vi "ReadHighTemp.vi"(8 "error in (no error)":errorcluster) -> (0 "error out":errorcluster, 1 "CurrentTemp(HighChamber)":dbl, 2 "CurrentTemp(HighChamber)":string)   [LabVIEW 2017, in "Thermal Shock.lvlib"]
uses:
  Thermal Shock.lvlib
  <vilib>/Instr/_visa.llb/VISA Configure Serial Port (Instr).vi
panel:
  in  "Stop":bool
  out "HighChamberSetPoint":dbl
  in  "Read Low Chamber!":bool
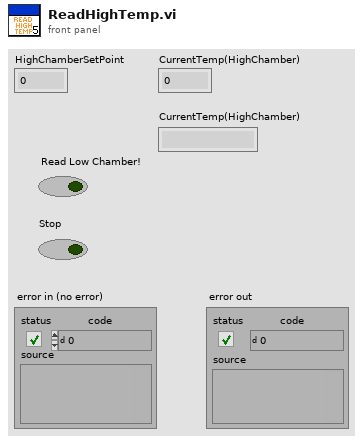
[diagram p1: front panel]
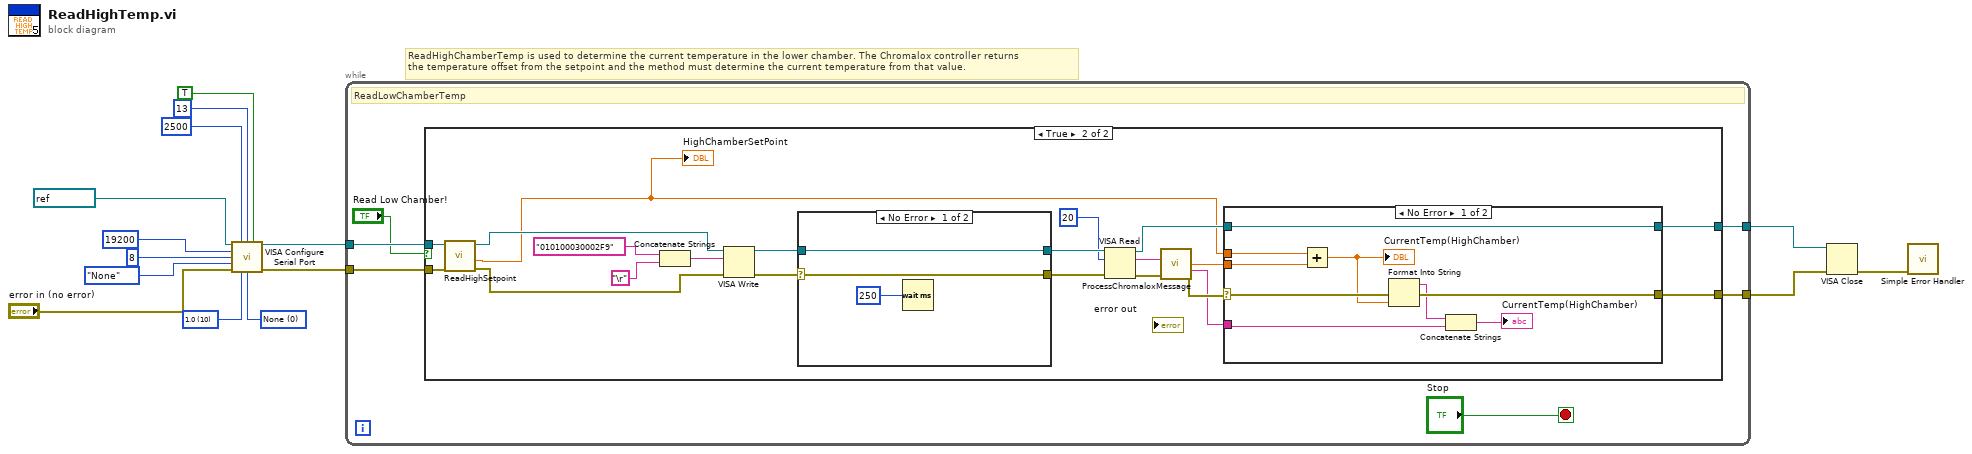
[diagram p0: block diagram]
diagram:
  w7 = u16 0 items=["None", "XON/XOFF", "RTS/CTS", "XON/XOFF & RTS/CTS", "DTR/DSR", "XON/XOFF & DTR/DSR"] ("flow control (0:none)")
  w9 = u16 10 items=["1.0"=10, "1.5"=15, "2.0"=20] ("stop bits (10: 1 bit)")
  # "ReadHighChamberTemp is used to determine the current temperature in the lower chamber. The Chromalox controller returns \nthe temperature offset from the setpoint and the method must determine the current temperature from that value."
  n1 = call-poly "VISA Configure Serial Port"("VISA resource name"=refnum<visa-resource-name> "COM1", "timeout (10sec)"=2500, "termination char\n(0xA = '\\n' = LF)"=u8 13, "Enable Termination\nChar (T)"=TRUE, "baud rate (9600)"=19200, "data bits (8)"=u16 8, "parity (0:none)"=enum16{"None", "Odd", "Even", "Mark", "Space"}."None", "error in (no error)"="error in (no error)", "stop bits (10: 1 bit)"=w9, "flow control (0:none)"=w7) -> ("VISA resource name out"=w5:refnum<visa-resource-name>, "error out"=w4:errorcluster)  [unwired: 4 in]
  n2 = while {
    tunnel: w5 -> [w20]
    tunnel: w4 -> [w19]
    tunnel: [w18] -> w3
    tunnel: [w17] -> w2
    stop <- "Stop" stop-if-true
    # "ReadLowChamberTemp"
    n3 = case shown="True" "Read Low Chamber!" {
      tunnel: w20 -> [w23 w24]
      tunnel: w19 -> [w22 w25]
      tunnel: [w22 w33] -> w18
      tunnel: [w23 w31] -> w17
      frame False {
      }
      frame True {
        n4 = call "ReadHighSetpoint.vi"("error in (no error)"=w25, "VISA resource name"=w24) -> ("error out"=w27:errorcluster, "HighChamberSetPoint"=w26:dbl, "VISA resource name out"=w28:refnum<visa-resource-name>)  [unwired: 6 in, 1 out]
        "HighChamberSetPoint" <- w26
        n5 = Concatenate Strings("010100030002F9", "\r") -> (w42:string)
        n6 = VISA Write(VISA resource name=w28, write buffer=w42, error in (no error)=w27) -> (VISA resource name out=w40:refnum<visa-resource-name>, error out=w41:errorcluster)  [unwired: 1 out]
        n7 = case shown="No Error" w41 {
          selector: w41 -> [w58 w59]
          tunnel: w40 -> [w57 w60]
          tunnel: [w58 w59] -> w38
          tunnel: [w57 w60] -> w39
          frame No Error {
            n8 = Wait (ms)(milliseconds to wait=250) -> ()  [unwired: 1 out]
          }
          frame Error {
          }
        }
        n9 = VISA Read(VISA resource name=w39, byte count=20, error in (no error)=w38) -> (VISA resource name out=w32:refnum<visa-resource-name>, read buffer=w36:string, error out=w35:errorcluster)  [unwired: 1 out]
        n10 = call "ProcessChromaloxMessage.vi"("Chromalox Message"=w36, "error in (no error)"=w35) -> ("Reading"=w29:dbl, "Units"=w30:string, "error out"=w34:errorcluster)  [unwired: 10 in, 1 out]
        n11 = case shown="No Error" w34 {
          selector: w34 -> [w52 w55]
          tunnel: w26 -> [w46 _]
          tunnel: [w51 w55] -> w33
          tunnel: w32 -> [w53 w54]
          tunnel: [w53 w54] -> w31
          tunnel: w30 -> [w48 _]
          tunnel: w29 -> [w45 _]
          frame No Error {
            n12 = Add(x=w46, y=w45) -> (x+y=w50:dbl)
            "CurrentTemp(HighChamber)" <- w50
            n13 = Format Into String(error in=w52, w50) -> (resulting string=w49:string, error out=w51:errorcluster)  [unwired: 2 in]
            n14 = Concatenate Strings(w49, w48) -> (→"CurrentTemp(HighChamber)":string)
          }
          frame Error {
          }
        }
      }
    }
  }
  n15 = VISA Close(VISA resource name=w2, error in (no error)=w3) -> (error out=w1:errorcluster)
  n16 = call <vilib>:"Simple Error Handler.vi"("error in (no error)"=w1) -> ()  [unwired: 4 in, 5 out]
